vi "PicoScope6000SetRapidSegments.vi"(5 "RapidBlock":bool, 7 "nSegments":u64 format="%.4p", 8 "error in (no error)":errorcluster, 11 "handle in":i16) -> (0 "error out":errorcluster, 3 "handle out":i16, 6 "nCaptures":u64)   [LabVIEW 2009]
doc: "Calls SetDataBuffers, and assigns Pico buffers"
uses:
  ps6000.dll
panel:
  out "nMaxSamples":u64
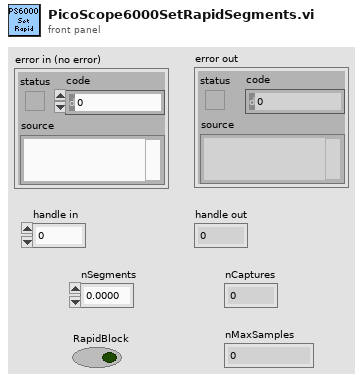
[diagram p1: front panel]
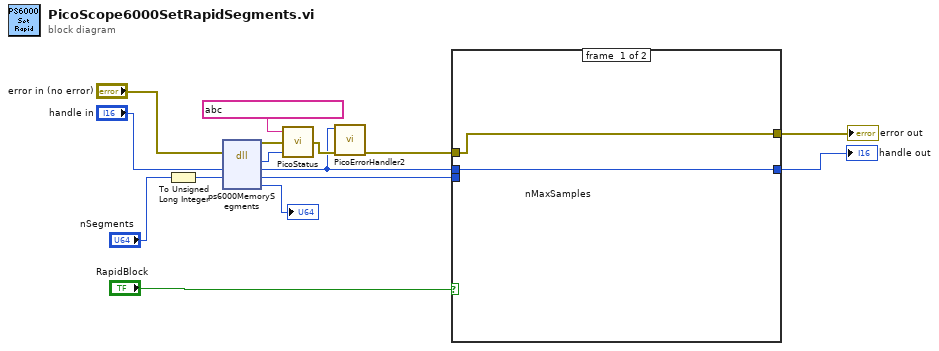
[diagram p0: block diagram]
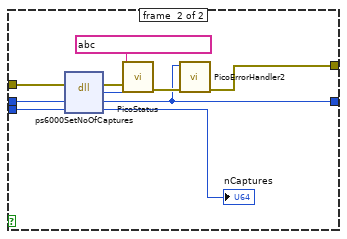
[diagram p2: hidden frame]
diagram:
  n1 = To Unsigned Long Integer(number="nSegments") -> (unsigned 32bit integer=w2:u32)
  n2 = dll-call lib="ps6000.dll" fn="ps6000MemorySegments" ("ps3000.dll:_ps3000_open_unit@0")(error in="error in (no error)", "handle"="handle in", "nSegments"=w2) -> (error out=w14:errorcluster, "PICO_STATUS"=w15:u32, "handle"=w10:i16, "nSegments"=w12:u32, "nMaxSamples"=→"nMaxSamples":u32)  [unwired: 3 in, 1 out]
  n3 = call "PicoStatus.vi"("PICO STATUS"=w15, "error in"=w14, "source"=string ?) -> ("error out"=w11:errorcluster)
  n4 = call "PicoErrorHandler2.vi"("error in (no error)"=w11, "handle In"=w10) -> ("error out"=w8:errorcluster)  [unwired: 9 in]
  n5 = case shown="True" "RapidBlock" {
    tunnel: w12 -> [_ w27]
    tunnel: w10 -> [w16 w24]
    tunnel: w8 -> [w17 w21]
    tunnel: [w17 w20] -> w5
    tunnel: [w16 w19] -> w4
    frame #0 {
    }
    frame #1 {
      n6 = dll-call lib="ps6000.dll" fn="ps6000SetNoOfCaptures" ("ps3000.dll:_ps3000_open_unit@0")(error in=w21, "handle"=w24, "nCaptures"=w27) -> (error out=w26:errorcluster, "PICO_STATUS"=w22:u32, "handle"=w19:i16, "nCaptures"=→"nCaptures":u32)  [unwired: 2 in, 1 out]
      n7 = call "PicoStatus.vi"("PICO STATUS"=w22, "error in"=w26, "source"=string ?) -> ("error out"=w23:errorcluster)
      n8 = call "PicoErrorHandler2.vi"("error in (no error)"=w23, "handle In"=w19) -> ("error out"=w20:errorcluster)  [unwired: 9 in]
    }
  }
  "error out" <- w5
  "handle out" <- w4
